vi "TDMS Advanced Synchronous Read.vi"() -> ()   [LabVIEW 2023]
doc: "This example demonstrates how to read data synchronously from a .tdms file using the Advanced TDMS VIs and functions."
panel:
  out "Waveform Graph":u32[](graph)
  # "Overview: Demonstrates the use of the Advanced TDMS functions to read a .tdms file synchronously.\nInstructions:\n1. Make sure you have already run TDMS Advanced Synchronous Write.vi.\n2. Run this VI.\n3. Delete the TDMS file (located at [LabVIEW Data]\\Example TDMS Advanced Synchronous Write.tdms) when you are done."
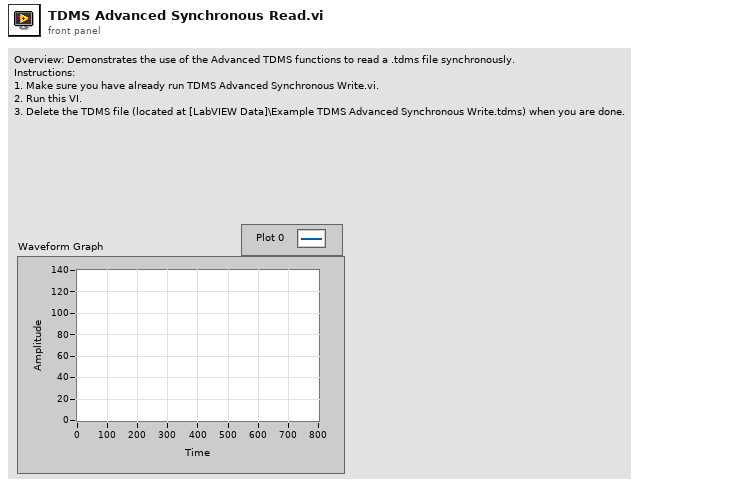
[diagram p1: front panel]
types:
  T1 = enum16{"open", "open or create", "create or replace", "create", "open (read-only)"}
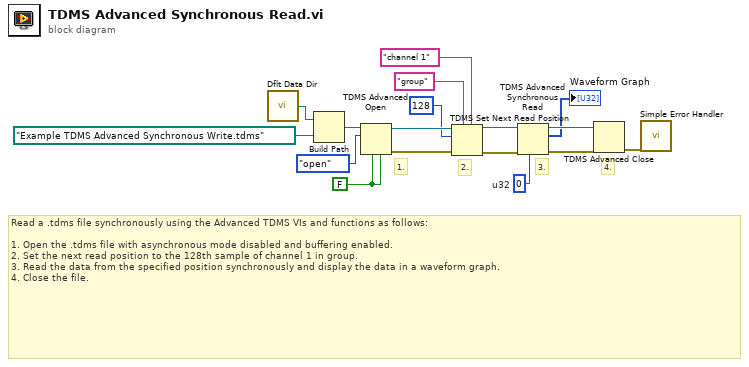
[diagram p0: block diagram]
diagram:
  w14 = FALSE ("enable asynchronous? (T)")
  w6 = u32 0  # u32
  # "Read a .tdms file synchronously using the Advanced TDMS VIs and functions as follows:\n\n1. Open the .tdms file with asynchronous mode disabled and buffering enabled.\n2. Set the next read position to the 128th sample of channel 1 in group.\n3. Read the data from the specified position synchronously and display the data in a waveform graph.\n4. Close the file."
  # "1."
  # "4."
  # "3."
  # "2."
  n1 = call <vilib>:"Dflt Data Dir.vi"() -> ("App:Default Data Directory"=w15:path)
  n2 = Build Path(base path=w15, name or relative path=path "Example TDMS Advanced Synchronous Write.tdms") -> (appended path=w17:path)
  n3 = TDMS Advanced Open(4:w14, 6:w14, 10:T1."open" ("operation (0:open)"), 11:w17) -> (0:w8:errorcluster, 3:w9:refnum<k34>)  [unwired: 1 in, 1 out]
  n4 = TDMS Set Next Read Position(5:"channel 1", 7:"group" ("group name (Untitled)"), 8:w8, 10:i64 128 ("offset (0)"), 11:w9) -> (0:w11:errorcluster, 3:w10:refnum<k34>)  [unwired: 1 in]
  n5 = TDMS Advanced Synchronous Read(6:w6, 8:w11, 11:w10) -> (0:w13:errorcluster, 2:→"Waveform Graph":u32[], 3:w12:refnum<k34>)  [unwired: 1 in, 1 out]
  n6 = TDMS Advanced Close(8:w13, 11:w12) -> (0:w2:errorcluster)  [unwired: 2 in, 1 out]
  n7 = call <vilib>:"Simple Error Handler.vi"("error in (no error)"=w2) -> ()  [unwired: 4 in, 5 out]
